vi "Template Action Test.vi"() -> ()   [LabVIEW 2014, in "Simple Sequencer TBM tests.lvlib"]
uses:
  <vilib>/NI/TBM Modules/Sequencer/testing/Simple Sequencer TBM tests.lvlib
  <vilib>/NI/TBM Modules/Sequencer/actions/template action/configuration/configuration data.ctl
  <vilib>/NI/TBM Modules/Sequencer/actions/template action/configuration/Template Action Config.lvclass
  <vilib>/NI/TBM Modules/Sequencer/actions/template action/configuration/Template Action Config.lvclass/Template Action Config.ctl
  <vilib>/NI/Tag Bus Module Framework/root configuration/TBM configuration.lvclass/TBM configuration.ctl
  <vilib>/NI/Tag Bus Module Framework/root configuration/Read instance name.vi
  <vilib>/NI/Tag Bus Module Framework/root configuration/create GUID.vi
panel:
  out "instance identifier 2":string
  out "instance identifier":string
  out "GUIDs equal?":bool
  out "Config. Data":T1
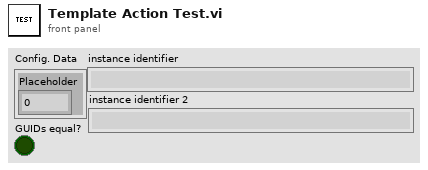
[diagram p1: front panel]
types:
  T1 = typedef "3D Gears Actions.lvlib/Template Action Config.lvclass/configuration data.ctl" = cluster{"Placeholder":dbl}
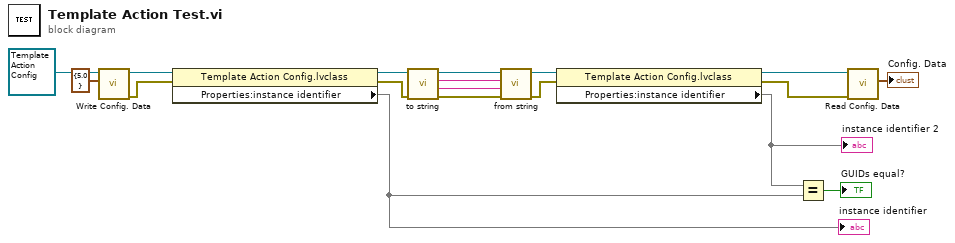
[diagram p0: block diagram]
diagram:
  n1 = call <vilib>:"Write Config. Data.vi"("Config. Data"=T1 {"Placeholder"=5.0}, "ActionCfg_Template Action in"=refnum<class "Template Action Config.lvclass"> refnum ("ActionCfg_Template Action.lvclass")) -> ("error out"=w6:errorcluster, "ActionCfg_Template Action out"=w11:refnum<class "Template Action Config.lvclass">)  [unwired: 8 in]
  n2 = property class="Template Action Config.lvclass"(reference=w11, error in=w6) -> (reference out=w7:refnum<class "Template Action Config.lvclass">, error out=w5:errorcluster, "Properties:instance identifier"=w9)
  "instance identifier" <- w9
  n3 = call-dynamic "to string.vi"("error in"=w5, "configuration in"=w7) -> ("error out"=w16:errorcluster, "data"=w14:string, "version"=w15:string, "configuration out"=w13:refnum<class "Template Action Config.lvclass">)  [unwired: 6 in]
  n4 = call-dynamic "from string.vi"("error in"=w16, "data"=w14, "version"=w15, "configuration in"=w13) -> ("error out"=w4:errorcluster, "configuration out"=w2:refnum<class "Template Action Config.lvclass">)  [unwired: 6 in]
  n5 = property class="Template Action Config.lvclass"(reference=w2, error in=w4) -> (reference out=w1:refnum<class "Template Action Config.lvclass">, error out=w3:errorcluster, "Properties:instance identifier"=w10)
  "instance identifier 2" <- w10
  n6 = Equal?(x=w10, y=w9) -> (x = y?=→"GUIDs equal?":bool)
  n7 = call <vilib>:"Read Config. Data.vi"("error in (no error)"=w3, "ActionCfg_Template Action in"=w1) -> ("Config. Data"=→"Config. Data":T1)  [unwired: 7 in, 2 out]
